vi "ProjectKFLOP.vi"() -> ()   [LabVIEW 2017]
uses:
  Control 1.ctl
  C:/KMotion434/KMotion/Release/KMotion_dotNet.dll
  Global 2.vi
panel:
  out "error out 3":errorcluster
  out "error out 2":errorcluster
  out "error out":errorcluster
  out "resulting string":string
  in  "Check_value":i32
  in  "BienLap":i32
  out "Status Check Done":dbl format="%11.1f"
  out "size":i32
  in  "Tab Control":enum32{"Manu", "Auto", "Setting"}(tab)
  in  "Add CheckDone":bool
  in  "Add Check":bool
  in  "Add Loop":bool
  in  "Test OUT":bool
  in  "Add Wait":bool
  in  "Add OUT":bool
  in  "TimeWait":dbl=5000.0
  in  "Value":dbl
  in  "Bit":dbl
  in  "Zero All":bool
  in  "Delele All":bool
  in  "Add Zero":bool
  in  "Add MoveXYZ":bool
  in  "Add Linear":bool
  in  "Save File":bool
  in  "Delete 1 Line":bool
  in  "Control":bool
  in  "Jog Speed":dbl=4000.0
  out "Vi Tri Save":string
  in  "file path (use dialog)":path
  out "Dest":dbl[](array[numeric])
  in  "Array Jog Command":dbl[](array[numeric])
  in  "V,A":dbl[](array[numeric]) caption="Dest 3"
  out "Auto":bool
  in  "Start":bool
  out "Value OUT":string
  out "Value Array":string[](array[string])
  out "Array":string[](array[string])
  out "Dest 2":T1
  out "Menu":bool
  in  "EMG":bool
  in  "Path":path
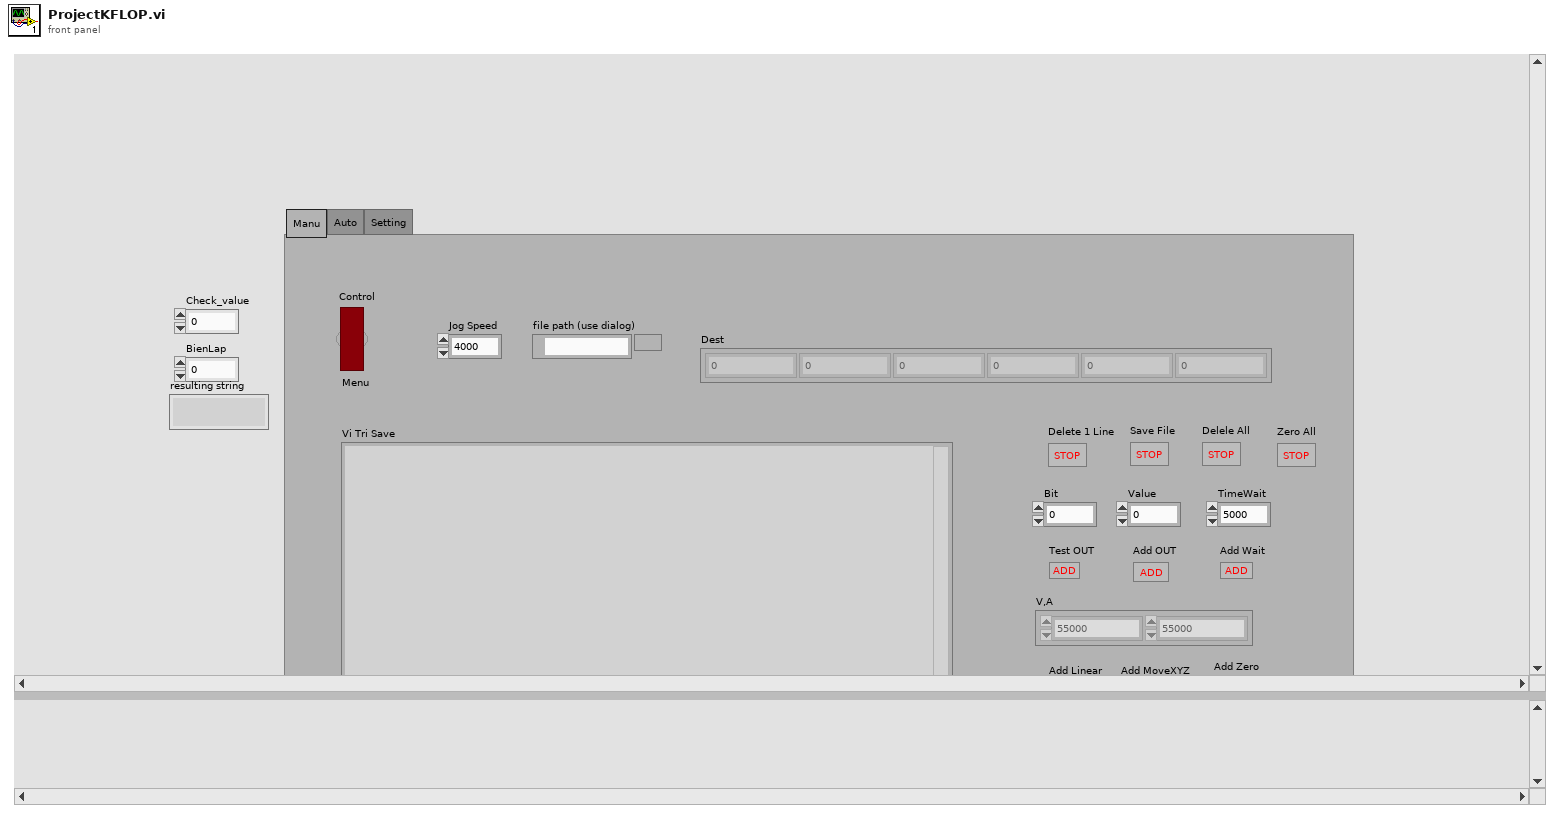
[diagram p1: front panel]
types:
  T1 = typedef "Control 1.ctl" = dbl[]
  T2 = cluster{"X":dbl, "Y":dbl, "Z":dbl, "A":dbl, "B":dbl, "C":dbl, "Numeric 7":dbl, "Numeric 8":dbl, "Numeric 9":dbl, "Numeric 10":dbl, "Numeric 11":dbl, "Numeric 12":dbl}
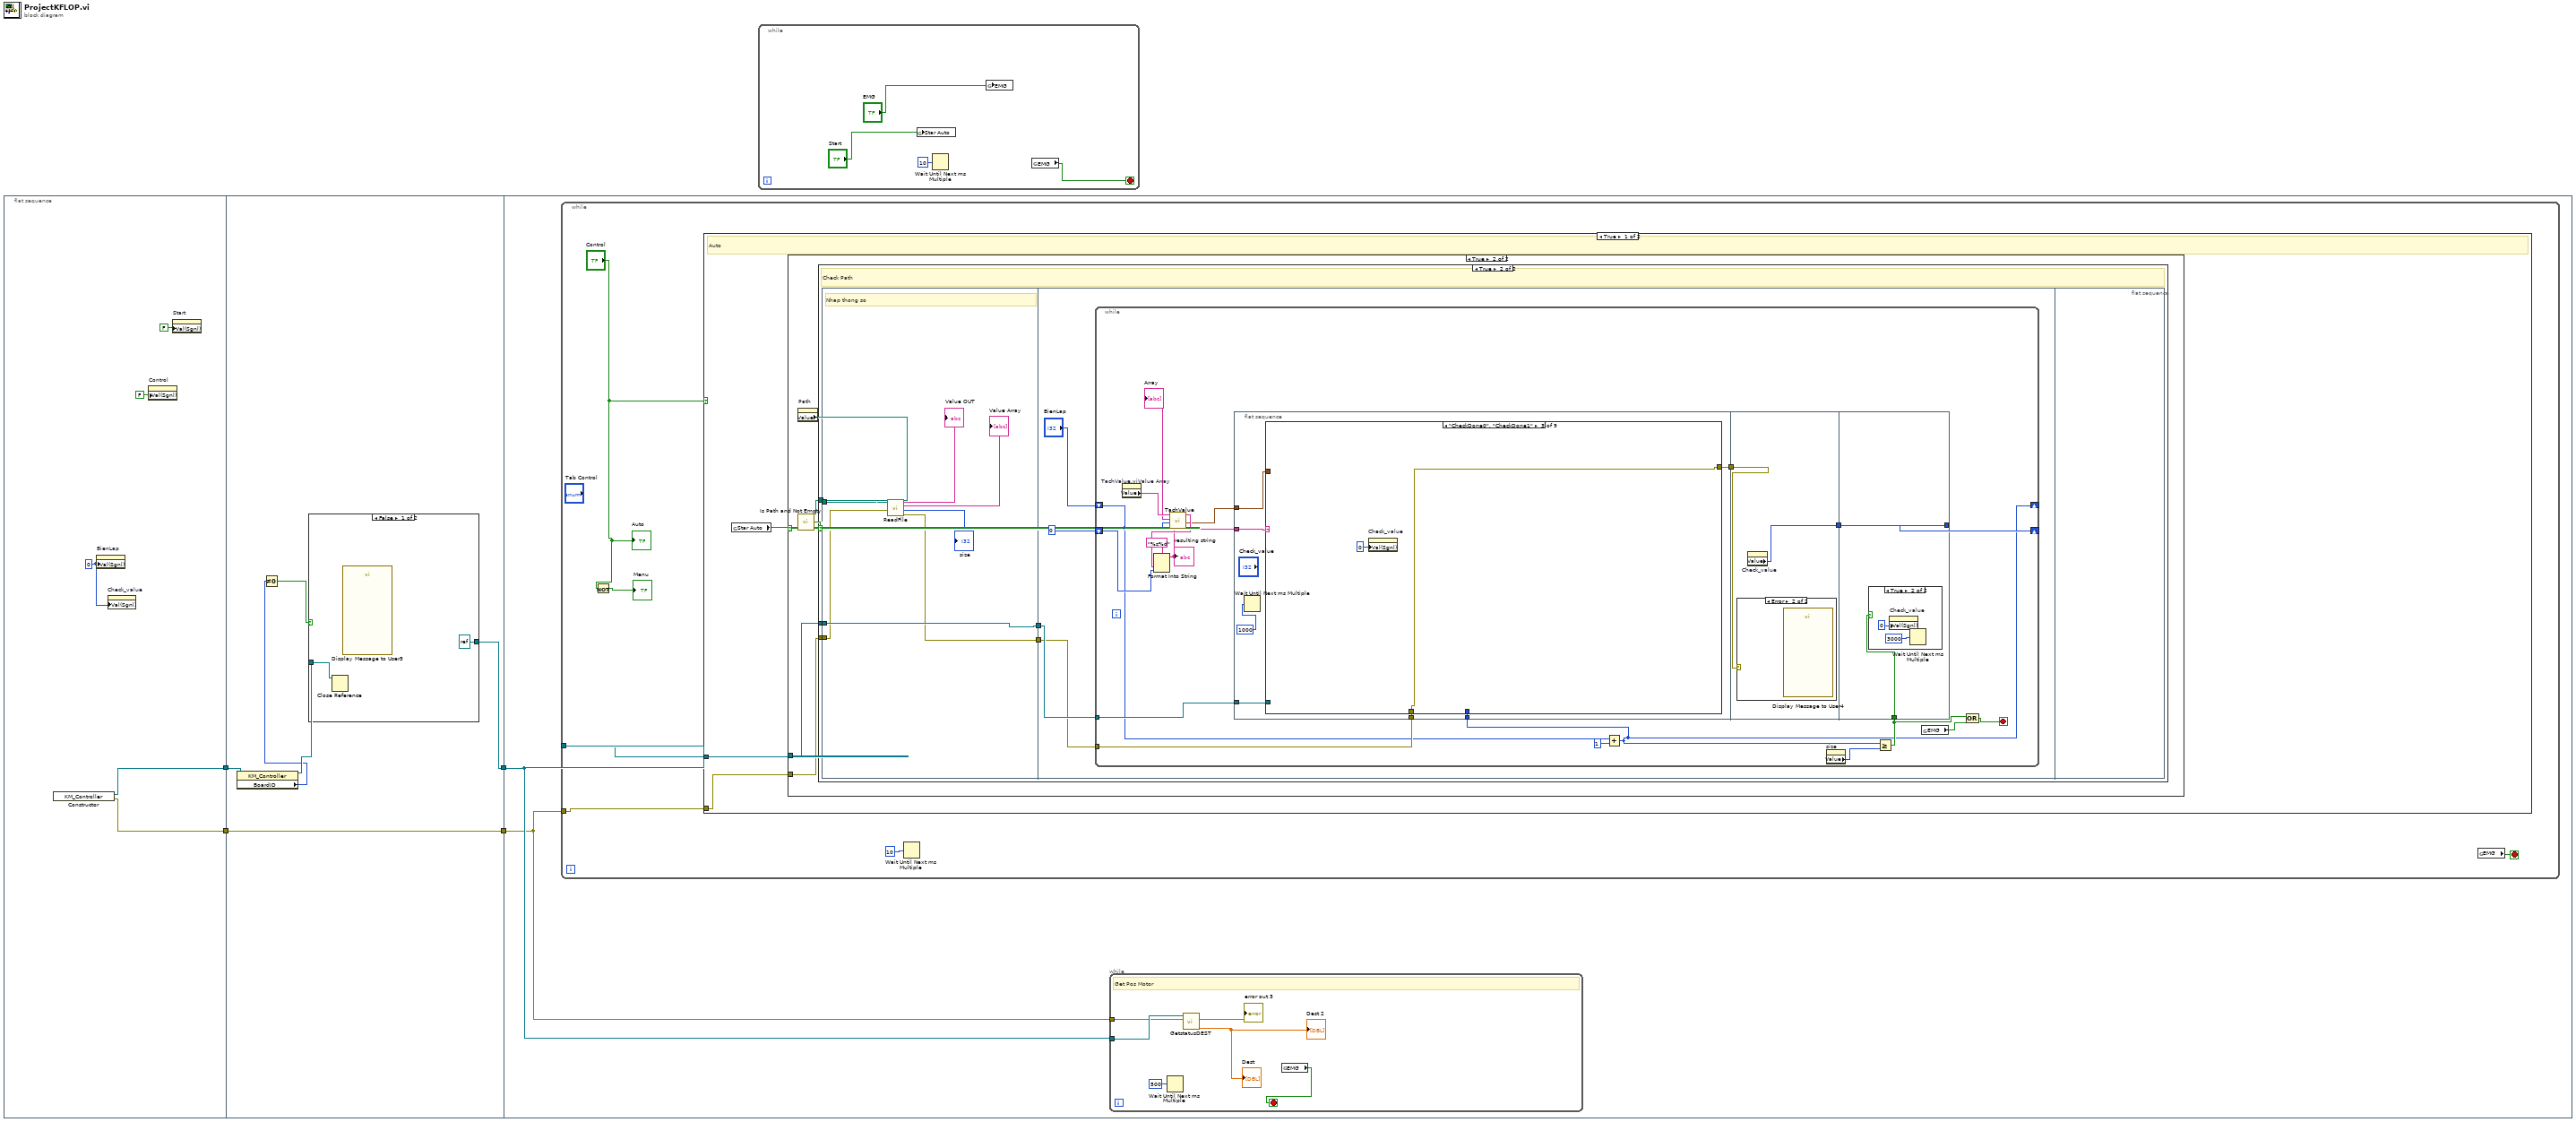
[diagram p0: block diagram]
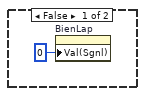
[diagram p3: hidden frame]
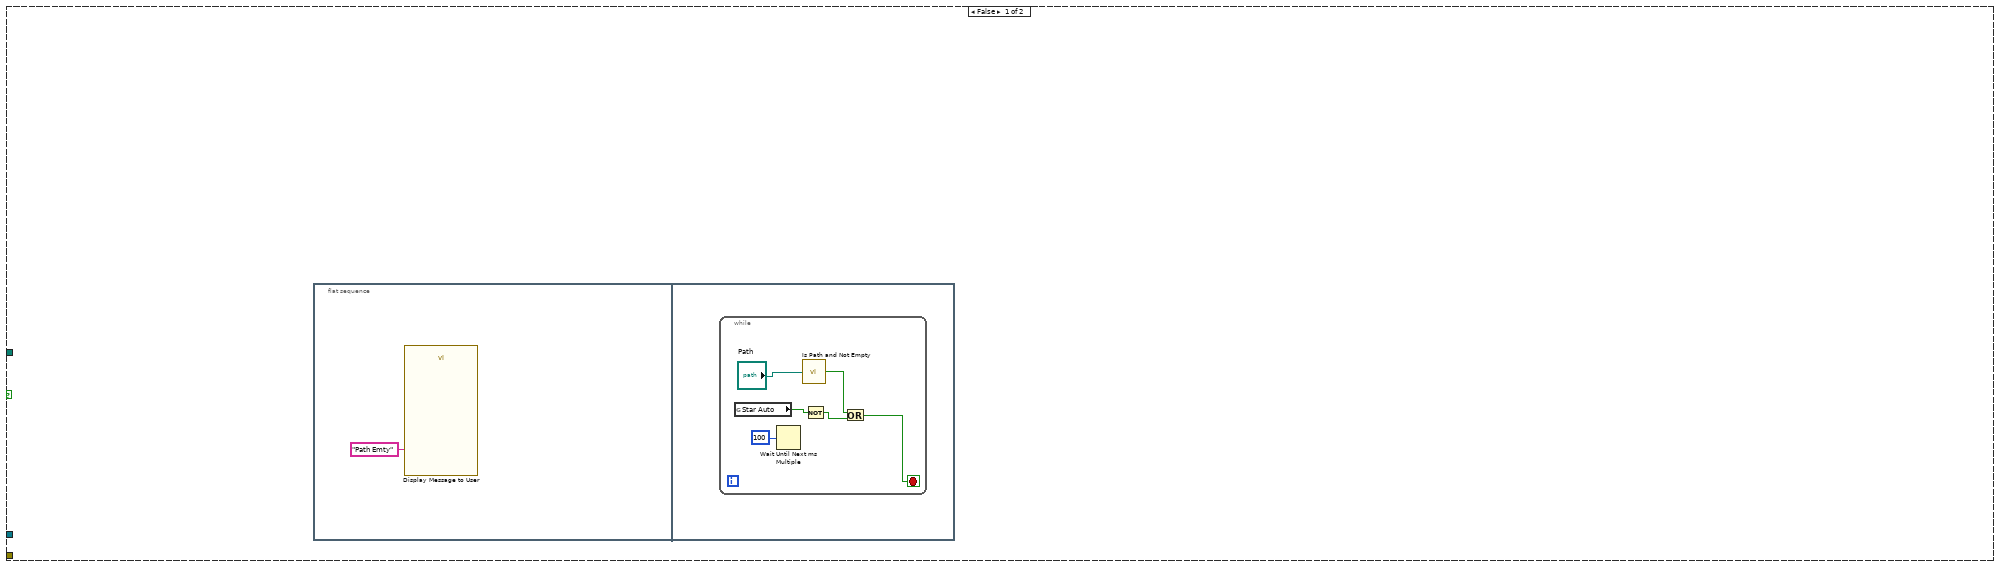
[diagram p4: hidden frame]
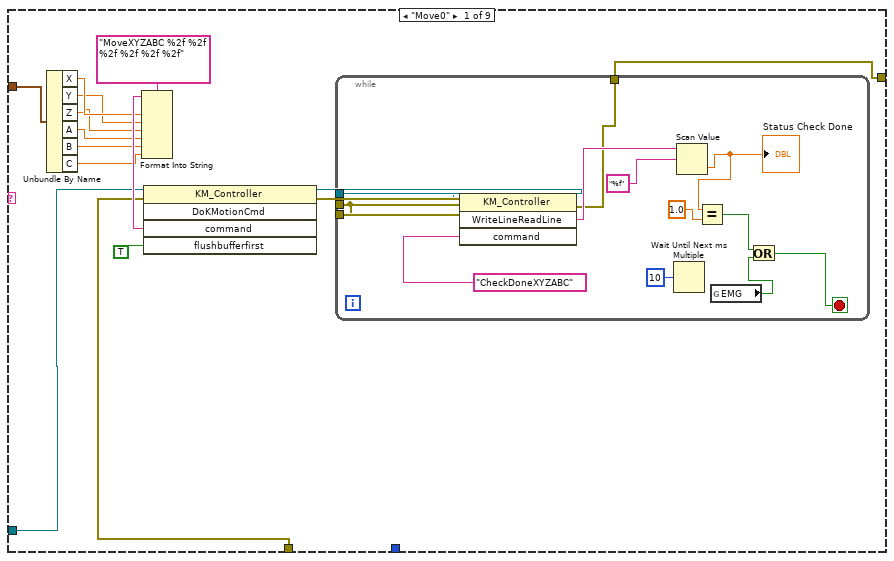
[diagram p5: hidden frame]
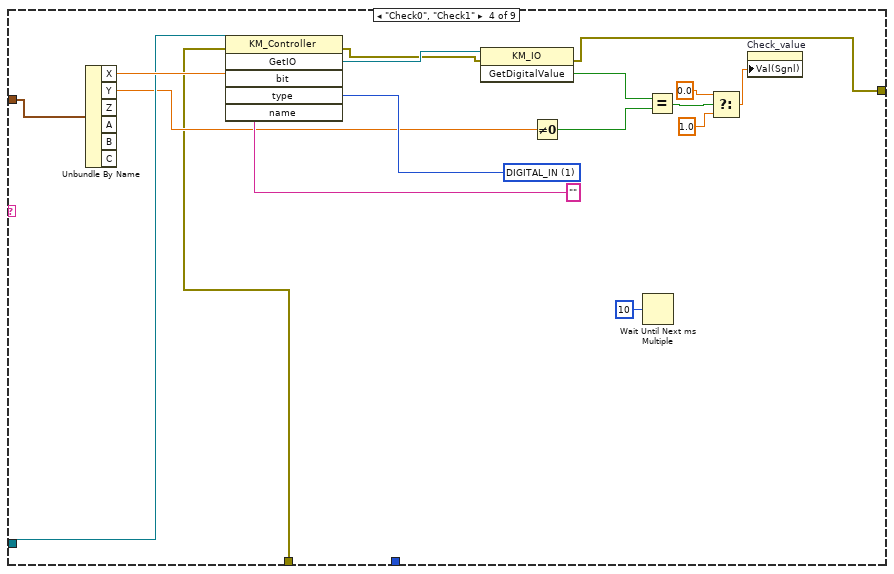
[diagram p7: hidden frame]
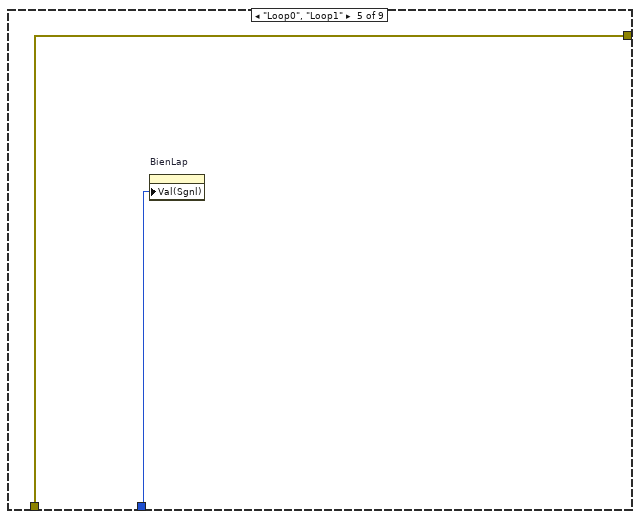
[diagram p8: hidden frame]
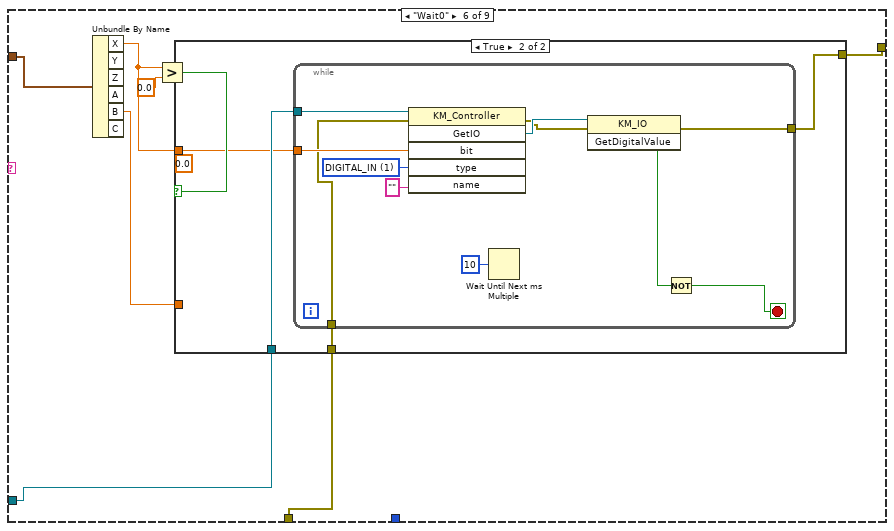
[diagram p9: hidden frame]
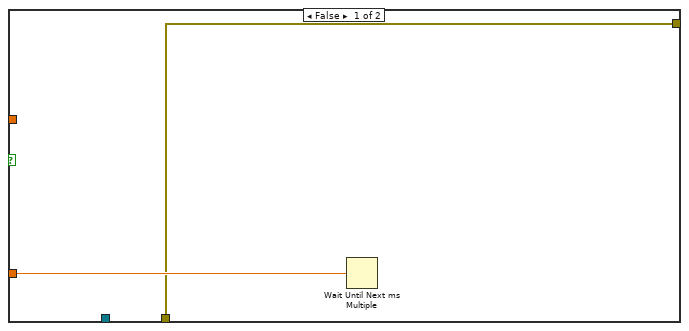
[diagram p10: hidden frame]
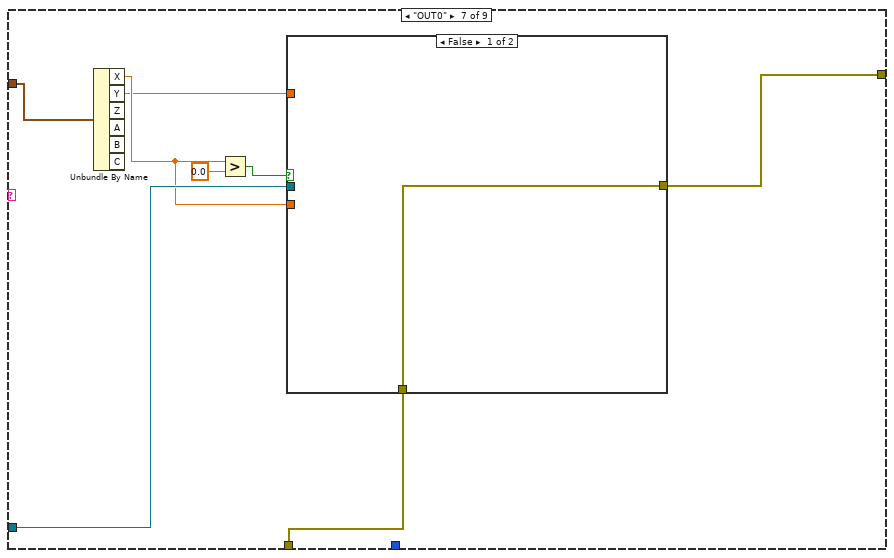
[diagram p11: hidden frame]
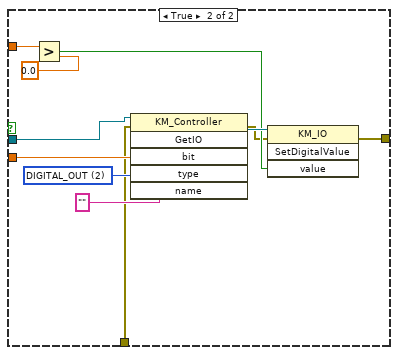
[diagram p12: hidden frame]
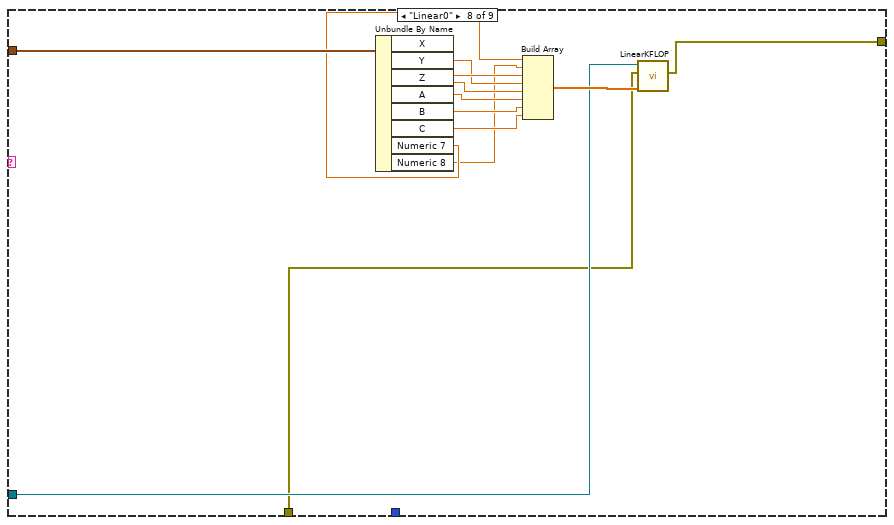
[diagram p13: hidden frame]
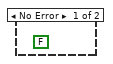
[diagram p15: hidden frame]
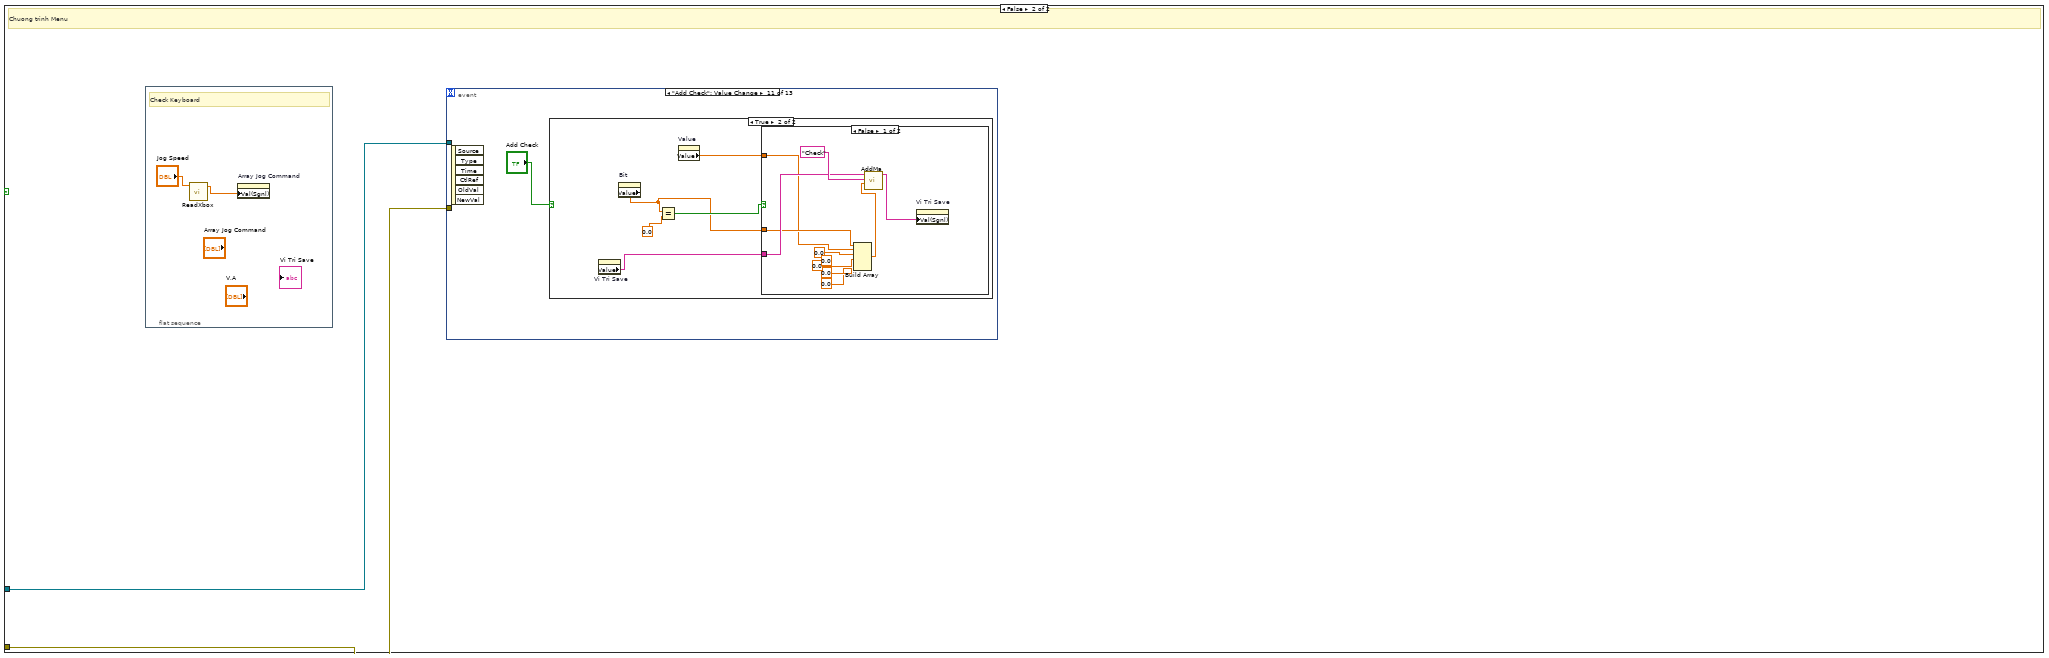
[diagram p17: hidden frame]
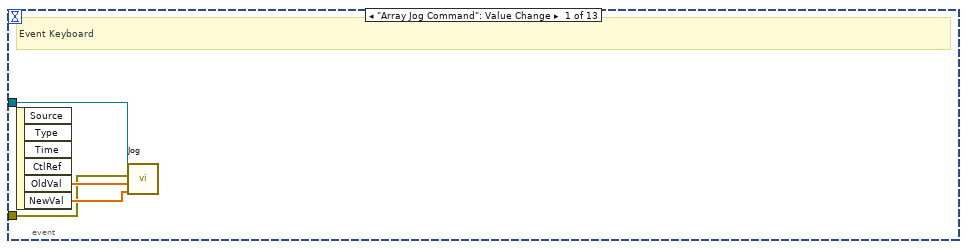
[diagram p18: hidden frame]
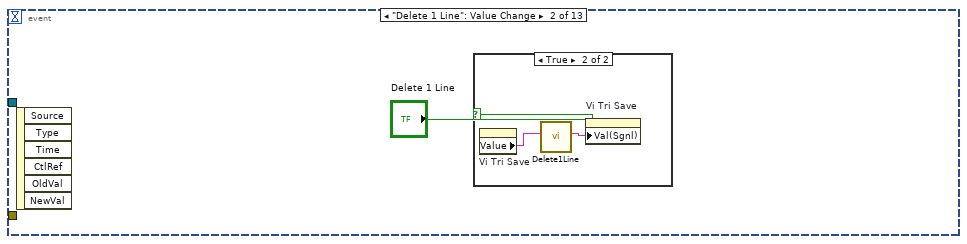
[diagram p19: hidden frame]
diagram:
  n1 = flat-sequence {
    tunnel: [w9] -> w2
    tunnel: [w8] -> w1
    tunnel: [w15] -> w4
    tunnel: [w14] -> w3
    tunnel: w2 -> [w13]
    tunnel: w1 -> [w15]
    tunnel: w4 -> [w19]
    tunnel: w3 -> [w20]
    frame #0 {
      w7 = 0 ("Value (Signaling)")
      n2 = constructor class="KM_Controller"() -> (reference out=w9:refnum<k24>, error out=w8:errorcluster)  [unwired: 3 in, 1 out]
      n3 = property on="BienLap" class="DigNum (strict)"("Val(Sgnl)"=w7) -> ()  [unwired: 2 in, 2 out]
      n4 = property on="Check_value" class="DigNum (strict)"("Val(Sgnl)"=w7) -> ()  [unwired: 2 in, 2 out]
      n5 = property on="Control" class="Bool (strict)"("Val(Sgnl)"=FALSE ("Value (Signaling)")) -> ()  [unwired: 2 in, 2 out]
      n6 = property on="Start" class="Bool (strict)"("Val(Sgnl)"=FALSE ("Value (Signaling)")) -> ()  [unwired: 2 in, 2 out]
    }
    frame #1 {
      n7 = property class="KM_Controller"(reference=w13) -> (reference out=w12:refnum<k24>, "BoardID"=w11:i32)  [unwired: 1 in, 1 out]
      n8 = Not Equal To 0?(x=w11) -> (x != 0?=w10:bool)
      n9 = case shown="False" w10 {
        tunnel: w12 -> [w16 w18]
        tunnel: [refnum<k24> refnum ("new reference") w18] -> w14
        frame False {
          n10 = Close Reference(reference=w16) -> ()  [unwired: 1 in, 1 out]
          n11 = call "Display Message to User3"() -> ()  [unwired: 10 in, 2 out]
        }
        frame True {
        }
      }
    }
    frame #2 {
      n12 = while {
        tunnel: w19 -> [w27]
        tunnel: w20 -> [w32]
        stop <- w28 stop-if-true
        n13 = Not(x="Control") -> (.not. x?=→"Menu":bool)
        n14 = case shown="True" "Control" {
          tunnel: w32 -> [w35 w204]
          tunnel: w27 -> [w33 w205]
          frame True {
            # "Auto"
            n15 = global read "Global 2.vi" "Star Auto"() -> (w34:bool)
            n16 = case shown="True" w34 {
              tunnel: w35 -> [_ w38]
              tunnel: w33 -> [_ w37]
              frame False {
                n17 = property on="BienLap" class="DigNum (strict)"("Val(Sgnl)"=0 ("Value (Signaling)")) -> ()  [unwired: 2 in, 2 out]
              }
              frame True {
                n18 = property on="Path" class="Path"() -> ("Value"=w39:path)  [unwired: 2 in, 2 out]
                n19 = call <vilib>:"Is Path and Not Empty.vi"("path"=w39) -> ("Is Path and Not Empty?"=w40:bool)  [unwired: 4 in]
                n20 = case shown="True" w40 {
                  tunnel: w39 -> [_ w51]
                  tunnel: w38 -> [_ w50]
                  tunnel: w37 -> [_ w49]
                  frame False {
                    n21 = flat-sequence {
                      frame #0 {
                        n22 = call "Display Message to User"("Message"="Path Emty") -> ()  [unwired: 9 in, 2 out]
                      }
                      frame #1 {
                        n23 = while {
                          stop <- w45 stop-if-true
                          n24 = global read "Global 2.vi" "Star Auto"() -> (w42:bool)
                          n25 = Wait Until Next ms Multiple(millisecond multiple=u32 100) -> ()  [unwired: 1 out]
                          n26 = call <vilib>:"Is Path and Not Empty.vi"("path"="Path") -> ("Is Path and Not Empty?"=w44:bool)  [unwired: 4 in]
                          n27 = Not(x=w42) -> (.not. x?=w43:bool)
                          n28 = Or(x=w44, y=w43) -> (x .or. y?=w45:bool)
                        }
                      }
                    }
                  }
                  frame True {
                    # "Check Path"
                    n29 = flat-sequence {
                      tunnel: [w55] -> w52
                      tunnel: w51 -> [w57]
                      tunnel: w50 -> [w55]
                      tunnel: w49 -> [w54]
                      tunnel: [w53] -> w48
                      tunnel: w52 -> [w63]
                      tunnel: w48 -> [w61]
                      frame #0 {
                        # "Nhap thong so"
                        n30 = call "ReadFile.vi"("error in"=w54, "Path"=w57) -> ("error out"=w53:errorcluster, "size"=→"size":i32, "Value Array"=→"Value Array":string[], "Value OUT"=→"Value OUT":string)  [unwired: 6 in]
                      }
                      frame #1 {
                        n31 = while {
                          shift-right: [w64] -> _
                          shift-left: "BienLap" -> [w65]
                          shift-right: [w70] -> _
                          shift-left: 0 -> [w79]
                          tunnel: w63 -> [w73]
                          tunnel: w61 -> [w72]
                          stop <- w75 stop-if-true
                          n32 = property on="TachValue.viValue Array" class="Arr (strict)"() -> ("Value"=w82:string[])  [unwired: 2 in, 2 out]
                          n33 = call "TachValue.vi"("index"=w65, "array"=w82) -> ("Cluster"=w69:T2, "Array"=→"Array":string[], "OUT First Value"=w77:string)  [unwired: 7 in]
                          n34 = Format Into String(format string="%s%d", w77, w79) -> (resulting string=w74:string)  [unwired: 2 in, 1 out]
                          "resulting string" <- w74
                          n35 = flat-sequence {
                            tunnel: w74 -> [w89]
                            tunnel: w69 -> [w88]
                            tunnel: w73 -> [w87]
                            tunnel: w72 -> [w86]
                            tunnel: [w85] -> w71
                            tunnel: w64 -> [w83]
                            tunnel: w71 -> [w199]
                            tunnel: [w198] -> w68
                            tunnel: [w201] -> w70
                            tunnel: w68 -> [w201]
                            tunnel: w67 -> [w200]
                            frame #0 {
                              n36 = Wait Until Next ms Multiple(millisecond multiple=u32 1000) -> ()  [unwired: 1 out]
                              n37 = case shown="\"CheckDone0\", \"CheckDone1\"" w89 {
                                tunnel: w88 -> [w99 _ _ w134 _ w146 w171 w196 _]
                                tunnel: w87 -> [w92 _ _ w135 _ w143 w168 w188 _]
                                tunnel: [w91 w117 w118 w121 w138 w139 w165 w185 w197] -> w85
                                tunnel: w86 -> [w90 w117 w118 w120 w138 w140 w164 w184 w197]
                                tunnel: w83 -> [_ _ _ _ w137 _ _ _ _]
                                frame "Move0" {
                                n38 = Unbundle By Name(w99) -> ("X"=w98:dbl, "Y"=w97:dbl, "Z"=w96:dbl, "A"=w95:dbl, "B"=w94:dbl, "C"=w93:dbl)
                                n39 = Format Into String(format string="MoveXYZABC %2f %2f %2f %2f %2f %2f", w98, w97, w96, w95, w94, w93) -> (resulting string=w102:string)  [unwired: 2 in, 1 out]
                                n40 = invoke class="KM_Controller" method="DoKMotionCmd"(reference=w92, error in=w90, "command"=w102, "flushbufferfirst"=TRUE) -> (reference out=w101:refnum<k24>, error out=w100:errorcluster)  [unwired: 1 in, 3 out]
                                n41 = while {
                                tunnel: [w107] -> _
                                tunnel: w101 -> [w108]
                                tunnel: w100 -> [w107]
                                tunnel: [w105] -> w91
                                stop <- w110 stop-if-true
                                n42 = invoke class="KM_Controller" method="WriteLineReadLine"(reference=w108, error in=w107, "command"="CheckDoneXYZABC") -> (error out=w105:errorcluster, "WriteLineReadLine"=w116:string)  [unwired: 1 in, 2 out]
                                n43 = Wait Until Next ms Multiple(millisecond multiple=u32 10) -> ()  [unwired: 1 out]
                                n44 = Scan Value(string=w116, format string="%f") -> (value=w113:dbl)  [unwired: 1 in, 1 out]
                                "Status Check Done" <- w113
                                n45 = Equal?(x=w113, y=1.0 ("x")) -> (x = y?=w109:bool)
                                n46 = global read "Global 2.vi" "EMG"() -> (w106:bool)
                                n47 = Or(x=w109, y=w106) -> (x .or. y?=w110:bool)
                                }
                                }
                                frame Default {
                                }
                                frame "CheckDone0", "CheckDone1" {
                                n48 = property on="Check_value" class="DigNum (strict)"("Val(Sgnl)"=0 ("Value (Signaling)")) -> ()  [unwired: 2 in, 2 out]
                                }
                                frame "Check0", "Check1" {
                                w133 = 1 items=["UNDEFINED", "DIGITAL_IN", "DIGITAL_OUT", "ANALOG_IN", "ANALOG_OUT"] ("type")
                                n49 = Unbundle By Name(w134) -> ("X"=w136:dbl, "Y"=w128:dbl)  [unwired: 4 out]
                                n50 = invoke class="KM_Controller" method="GetIO"(reference=w135, error in=w120, "bit"=w136, "type"=w133, "name"="") -> (error out=w122:errorcluster, "GetIO"=w132:refnum<k24>)  [unwired: 1 in, 4 out]
                                n51 = invoke class="KM_IO" method="GetDigitalValue"(reference=w132, error in=w122) -> (error out=w121:errorcluster, "GetDigitalValue"=w129:bool)  [unwired: 1 in, 1 out]
                                n52 = Not Equal To 0?(x=w128) -> (x != 0?=w127:bool)
                                n53 = Wait Until Next ms Multiple(millisecond multiple=u32 10) -> ()  [unwired: 1 out]
                                n54 = Equal?(x=w129, y=w127) -> (x = y?=w123:bool)
                                n55 = Select(t=0.0, s=w123, f=1.0) -> (s? t:f=w126:dbl)
                                n56 = property on="Check_value" class="DigNum (strict)"("Val(Sgnl)"=w126) -> ()  [unwired: 2 in, 2 out]
                                }
                                frame "Loop0", "Loop1" {
                                n57 = property on="BienLap" class="DigNum (strict)"("Val(Sgnl)"=w137) -> ()  [unwired: 2 in, 2 out]
                                }
                                frame "Wait0" {
                                n58 = Unbundle By Name(w146) -> ("X"=w142:dbl, "B"=w145:dbl)  [unwired: 4 out]
                                n59 = Greater?(x=w142, y=0.0) -> (0:w141:bool)
                                n60 = case shown="True" w141 {
                                tunnel: w145 -> [w148 _]
                                tunnel: w143 -> [_ w152]
                                tunnel: w142 -> [_ w151]
                                tunnel: [w147 w150] -> w139
                                tunnel: w140 -> [w147 w149]
                                frame False {
                                n61 = Wait Until Next ms Multiple(millisecond multiple=w148) -> ()  [unwired: 1 out]
                                }
                                frame True {
                                (unwired) 0.0 ("y")
                                n62 = while {
                                tunnel: w152 -> [w163]
                                tunnel: w151 -> [w161]
                                tunnel: [w154] -> w150
                                tunnel: w149 -> [w153]
                                stop <- w158 stop-if-true
                                w162 = 1 items=["UNDEFINED", "DIGITAL_IN", "DIGITAL_OUT", "ANALOG_IN", "ANALOG_OUT"] ("type")
                                n63 = invoke class="KM_Controller" method="GetIO"(reference=w163, error in=w153, "bit"=w161, "type"=w162, "name"="") -> (error out=w155:errorcluster, "GetIO"=w160:refnum<k24>)  [unwired: 1 in, 4 out]
                                n64 = Wait Until Next ms Multiple(millisecond multiple=u32 10) -> ()  [unwired: 1 out]
                                n65 = invoke class="KM_IO" method="GetDigitalValue"(reference=w160, error in=w155) -> (error out=w154:errorcluster, "GetDigitalValue"=w157:bool)  [unwired: 1 in, 1 out]
                                n66 = Not(x=w157) -> (.not. x?=w158:bool)
                                }
                                }
                                }
                                }
                                frame "OUT0" {
                                n67 = Unbundle By Name(w171) -> ("X"=w167:dbl, "Y"=w166:dbl)  [unwired: 4 out]
                                n68 = Greater?(x=w167, y=0.0) -> (0:w170:bool)
                                n69 = case shown="False" w170 {
                                tunnel: w168 -> [_ w176]
                                tunnel: w167 -> [_ w177]
                                tunnel: w166 -> [_ w180]
                                tunnel: [w172 w174] -> w165
                                tunnel: w164 -> [w172 w173]
                                frame False {
                                }
                                frame True {
                                w183 = 2 items=["UNDEFINED", "DIGITAL_IN", "DIGITAL_OUT", "ANALOG_IN", "ANALOG_OUT"] ("type")
                                n70 = Greater?(x=w180, y=0.0) -> (0:w179:bool)
                                n71 = invoke class="KM_Controller" method="GetIO"(reference=w176, error in=w173, "bit"=w177, "type"=w183, "name"="") -> (error out=w175:errorcluster, "GetIO"=w181:refnum<k24>)  [unwired: 1 in, 4 out]
                                n72 = invoke class="KM_IO" method="SetDigitalValue"(reference=w181, error in=w175, "value"=w179) -> (error out=w174:errorcluster)  [unwired: 1 in, 3 out]
                                }
                                }
                                }
                                frame "Linear0" {
                                n73 = Unbundle By Name(w196) -> ("X"=w195:dbl, "Y"=w194:dbl, "Z"=w193:dbl, "A"=w192:dbl, "B"=w191:dbl, "C"=w190:dbl, "Numeric 7"=w187:dbl, "Numeric 8"=w186:dbl)
                                n74 = Build Array(w187, w186, w195, w194, w193, w192, w191, w190) -> (w189:dbl[])
                                n75 = call "LinearKFLOP.vi"("Array"=w189, "error in (no error)"=w184, "new reference"=w188) -> ("error out"=w185:errorcluster)  [unwired: 7 in, 1 out]
                                }
                                frame "M010" {
                                }
                              }
                            }
                            frame #1 {
                              n76 = case shown="Error" w199 {
                                frame No Error {
                                (unwired) FALSE ("OK")
                                }
                                frame Error {
                                n77 = call "Display Message to User4"() -> ()  [unwired: 10 in, 2 out]
                                }
                              }
                              n78 = property on="Check_value" class="DigNum (strict)"() -> ("Value"=w198:i32)  [unwired: 2 in, 2 out]
                            }
                            frame #2 {
                              n79 = case shown="True" w200 {
                                frame False {
                                }
                                frame True {
                                n80 = property on="Check_value" class="DigNum (strict)"("Val(Sgnl)"=0 ("Value (Signaling)")) -> ()  [unwired: 2 in, 2 out]
                                n81 = Wait Until Next ms Multiple(millisecond multiple=u32 3000) -> ()  [unwired: 1 out]
                                }
                              }
                            }
                          }
                          n82 = Add(x=w65, y=1) -> (x+y=w64:i32)
                          n83 = property on="size" class="DigNum (strict)"() -> ("Value"=w66:i32)  [unwired: 2 in, 2 out]
                          n84 = Greater Or Equal?(x=w64, y=w66) -> (x >= y?=w67:bool)
                          n85 = global read "Global 2.vi" "EMG"() -> (w76:bool)
                          n86 = Compound Arithmetic op=OR(w67, w76) -> (w75:bool)
                        }
                      }
                      frame #2 {
                      }
                    }
                  }
                }
              }
            }
          }
          frame False {
            # "Chuong trinh Menu"
            n87 = flat-sequence {
              frame #0 {
                # "Check Keyboard"
                n88 = call "ReadXbox.vi"("Jog Speed"="Jog Speed") -> ("Array Jog Command"=w312:dbl[])  [unwired: 5 in]
                n89 = property on="Array Jog Command" class="Arr (strict)"("Val(Sgnl)"=w312) -> ()  [unwired: 2 in, 2 out]
              }
            }
            n90 = event shown="[10] \"Add Check\": Value Change" {
              selector: _ -> [_ _ _ _ _ _ _ _ _ _ _ _ _]
              dyn-events: _ -> [_ _ _ _ _ _ _ _ _ _ _ _ _]
              timeout: _ -> [_ _ _ _ _ _ _ _ _ _ _ _ _]
              tunnel: w204 -> [w207 _ _ _ w218 w234 _ _ _ _ _ _ _]
              tunnel: w205 -> [w206 _ _ _ w219 w232 _ _ _ _ _ _ _]
              event "Array Jog Command": Value Change {
                # "Event Keyboard"
                n91 = event-data() -> ("OldVal"=w209:dbl[], "NewVal"=w208:dbl[])  [unwired: 1 in, 4 out]
                n92 = call "Jog.vi"("NewVal"=w208, "Old Var"=w209, "error in (no error)"=w206, "reference"=w207) -> ()  [unwired: 6 in, 2 out]
              }
              event "Delete 1 Line": Value Change {
                n93 = event-data() -> ()  [unwired: 1 in, 6 out]
                n94 = case shown="True" "Delete 1 Line" {
                  frame False {
                  }
                  frame True {
                    n95 = property on="Vi Tri Save" class="Str"() -> ("Value"=w212:string)  [unwired: 2 in, 2 out]
                    n96 = call "Delete1Line.vi"("Value"=w212) -> ("String"=w211:string)  [unwired: 10 in]
                    n97 = property on="Vi Tri Save" class="Str"("Val(Sgnl)"=w211) -> ()  [unwired: 2 in, 2 out]
                  }
                }
              }
              event "Delele All": Value Change {
                n98 = event-data() -> ()  [unwired: 1 in, 6 out]
                n99 = case shown="True" "Delele All" {
                  frame False {
                  }
                  frame True {
                    n100 = property on="Vi Tri Save" class="Str"("Val(Sgnl)"="" ("Value (Signaling)")) -> ()  [unwired: 2 in, 2 out]
                  }
                }
              }
              event "Save File": Value Change {
                n101 = event-data() -> ()  [unwired: 1 in, 6 out]
                n102 = case shown="True" "Save File" {
                  frame False {
                  }
                  frame True {
                    n103 = property on="Vi Tri Save" class="Str"() -> ("Value"=w216:string)  [unwired: 2 in, 2 out]
                    n104 = call "SaveFile.vi"("text"=w216, "file path (use dialog)"="file path (use dialog)") -> ()  [unwired: 10 in]
                  }
                }
              }
              event "Test OUT": Value Change {
                n105 = event-data() -> ()  [unwired: 1 in, 6 out]
                n106 = case shown="True" "Test OUT" {
                  tunnel: w218 -> [_ w224]
                  tunnel: w219 -> [_ w223]
                  frame False {
                  }
                  frame True {
                    w231 = 2 items=["UNDEFINED", "DIGITAL_IN", "DIGITAL_OUT", "ANALOG_IN", "ANALOG_OUT"] ("type")
                    n107 = property on="Value" class="DigNum (strict)"() -> ("Value"=w226:dbl)  [unwired: 2 in, 2 out]
                    n108 = Greater?(x=w226, y=0.0) -> (0:w228:bool)
                    n109 = property on="Bit" class="DigNum (strict)"() -> ("Value"=w225:dbl)  [unwired: 2 in, 2 out]
                    n110 = invoke class="KM_Controller" method="GetIO"(reference=w224, error in=w223, "bit"=w225, "type"=w231, "name"="") -> (error out=w222:errorcluster, "GetIO"=w229:refnum<k24>)  [unwired: 1 in, 4 out]
                    n111 = invoke class="KM_IO" method="SetDigitalValue"(reference=w229, error in=w222, "value"=w228) -> (error out=→"error out":errorcluster)  [unwired: 1 in, 3 out]
                  }
                }
              }
              event "Zero All": Value Change {
                n112 = event-data() -> ()  [unwired: 1 in, 6 out]
                n113 = case shown="True" "Zero All" {
                  tunnel: w234 -> [_ w237]
                  tunnel: w232 -> [_ w236]
                  frame False {
                  }
                  frame True {
                    n114 = call "SetZeroALL.vi"("error in (no error)"=w236, "reference"=w237) -> ("error out"=→"error out 2":errorcluster)  [unwired: 8 in, 1 out]
                  }
                }
              }
              event "Add Zero": Value Change {
                n115 = event-data() -> ()  [unwired: 1 in, 6 out]
                n116 = case shown="True" "Add Zero" {
                  frame False {
                  }
                  frame True {
                    n117 = property on="V,A" class="Arr (strict)"() -> ("Value"=w240:dbl[])  [unwired: 2 in, 2 out]
                    n118 = property on="Vi Tri Save" class="Str"() -> ("Value"=w242:string)  [unwired: 2 in, 2 out]
                    n119 = call "AddMa.vi"("Dest 3"=w240, "Toa Do"=dbl[] [], "MaBegin"="Linear", "String IN"=w242) -> ("String OUT"=w241:string)  [unwired: 7 in]
                    n120 = property on="Vi Tri Save" class="Str"("Val(Sgnl)"=w241) -> ()  [unwired: 2 in, 2 out]
                  }
                }
              }
              event "Add OUT": Value Change {
                n121 = event-data() -> ()  [unwired: 1 in, 6 out]
                n122 = property on="Bit" class="DigNum (strict)"() -> ("Value"=w246:dbl)  [unwired: 2 in, 2 out]
                n123 = case shown="True" "Add OUT" {
                  tunnel: w246 -> [_ w252]
                  tunnel: "Value" -> [_ w251]
                  frame False {
                  }
                  frame True {
                    n124 = Build Array(w252, w251, 0.0 ("element"), 0.0 ("element"), 0.0 ("element"), 0.0 ("element")) -> (w255:dbl[])
                    n125 = property on="Vi Tri Save" class="Str"() -> ("Value"=w253:string)  [unwired: 2 in, 2 out]
                    n126 = call "AddMa.vi"("Toa Do"=w255, "MaBegin"="OUT", "String IN"=w253) -> ("String OUT"=w254:string)  [unwired: 8 in]
                    n127 = property on="Vi Tri Save" class="Str"("Val(Sgnl)"=w254) -> ()  [unwired: 2 in, 2 out]
                  }
                }
              }
              event "Add Wait": Value Change {
                n128 = event-data() -> ()  [unwired: 1 in, 6 out]
                n129 = case shown="True" "Add Wait" {
                  tunnel: "Bit" -> [_ w265]
                  tunnel: "TimeWait" -> [_ w264]
                  frame False {
                  }
                  frame True {
                    n130 = Build Array(w265, 0.0 ("element"), 0.0 ("element"), 0.0 ("element"), w264, 0.0 ("element")) -> (w266:dbl[])
                    n131 = property on="Vi Tri Save" class="Str"() -> ("Value"=w269:string)  [unwired: 2 in, 2 out]
                    n132 = call "AddMa.vi"("Toa Do"=w266, "MaBegin"="Wait", "String IN"=w269) -> ("String OUT"=w268:string)  [unwired: 8 in]
                    n133 = property on="Vi Tri Save" class="Str"("Val(Sgnl)"=w268) -> ()  [unwired: 2 in, 2 out]
                  }
                }
              }
              event "Add Loop": Value Change {
                n134 = event-data() -> ()  [unwired: 1 in, 6 out]
                n135 = case shown="True" "Add Loop" {
                  frame False {
                  }
                  frame True {
                    n136 = property on="Vi Tri Save" class="Str"() -> ("Value"=w279:string)  [unwired: 2 in, 2 out]
                    n137 = Build Array(0.0 ("element"), 0.0 ("element"), 0.0 ("element"), 0.0 ("element"), 0.0 ("element"), 0.0 ("element")) -> (w271:dbl[])
                    n138 = call "AddMa.vi"("Toa Do"=w271, "MaBegin"="Loop", "String IN"=w279) -> ("String OUT"=w280:string)  [unwired: 8 in]
                    n139 = property on="Vi Tri Save" class="Str"("Val(Sgnl)"=w280) -> ()  [unwired: 2 in, 2 out]
                  }
                }
              }
              event "Add Check": Value Change {
                n140 = event-data() -> ()  [unwired: 1 in, 6 out]
                n141 = case shown="True" "Add Check" {
                  frame False {
                  }
                  frame True {
                    n142 = property on="Vi Tri Save" class="Str"() -> ("Value"=w282:string)  [unwired: 2 in, 2 out]
                    n143 = property on="Bit" class="DigNum (strict)"() -> ("Value"=w284:dbl)  [unwired: 2 in, 2 out]
                    n144 = Equal?(x=w284, y=0.0) -> (x = y?=w285:bool)
                    n145 = property on="Value" class="DigNum (strict)"() -> ("Value"=w283:dbl)  [unwired: 2 in, 2 out]
                    n146 = case shown="False" w285 {
                      tunnel: w282 -> [w291 _]
                      tunnel: w284 -> [w289 _]
                      tunnel: w283 -> [w288 _]
                      frame False {
                        (unwired) 0.0 ("element")
                        n147 = Build Array(w289, w288, 0.0 ("element"), 0.0 ("element"), 0.0 ("element"), 0.0 ("element")) -> (w287:dbl[])
                        n148 = call "AddMa.vi"("Toa Do"=w287, "MaBegin"="Check", "String IN"=w291) -> ("String OUT"=w290:string)  [unwired: 8 in]
                        n149 = property on="Vi Tri Save" class="Str"("Val(Sgnl)"=w290) -> ()  [unwired: 2 in, 2 out]
                      }
                      frame True {
                        n150 = call "Display Message to User2"() -> ()  [unwired: 10 in, 2 out]
                      }
                    }
                  }
                }
              }
              event "Add CheckDone": Value Change {
                n151 = event-data() -> ()  [unwired: 1 in, 6 out]
                n152 = case shown="True" "Add CheckDone" {
                  frame False {
                  }
                  frame True {
                    n153 = property on="Vi Tri Save" class="Str"() -> ("Value"=w299:string)  [unwired: 2 in, 2 out]
                    n154 = call "AddMa.vi"("MaBegin"="CheckDone", "String IN"=w299) -> ("String OUT"=w300:string)  [unwired: 9 in]
                    n155 = property on="Vi Tri Save" class="Str"("Val(Sgnl)"=w300) -> ()  [unwired: 2 in, 2 out]
                  }
                }
              }
              event "Add Linear", "Add MoveXYZ": Value Change {
                n156 = event-data() -> ()  [unwired: 1 in, 6 out]
                n157 = Select(t="Move", s="Add MoveXYZ", f="Linear") -> (s? t:f=w301:string)
                n158 = Or(x="Add Linear", y="Add MoveXYZ") -> (x .or. y?=w302:bool)
                n159 = case shown="True" w302 {
                  tunnel: w301 -> [_ w308]
                  frame False {
                  }
                  frame True {
                    n160 = property on="Vi Tri Save" class="Str"() -> ("Value"=w310:string)  [unwired: 2 in, 2 out]
                    n161 = property on="Dest" class="Arr (strict)"() -> ("Value"=w309:dbl[])  [unwired: 2 in, 2 out]
                    n162 = property on="V,A" class="Arr (strict)"() -> ("Value"=w307:dbl[])  [unwired: 2 in, 2 out]
                    n163 = call "AddMa.vi"("Dest 3"=w307, "Toa Do"=w309, "MaBegin"=w308, "String IN"=w310) -> ("String OUT"=w311:string)  [unwired: 7 in]
                    n164 = property on="Vi Tri Save" class="Str"("Val(Sgnl)"=w311) -> ()  [unwired: 2 in, 2 out]
                  }
                }
              }
            }
          }
        }
        n165 = Wait Until Next ms Multiple(millisecond multiple=u32 10) -> ()  [unwired: 1 out]
        n166 = global read "Global 2.vi" "EMG"() -> (w28:bool)
        "Auto" <- "Control"
      }
      n167 = while {
        tunnel: w20 -> [w25]
        tunnel: w19 -> [w22]
        stop <- w23 stop-if-true
        # "Get Pos Motor"
        n168 = Wait Until Next ms Multiple(millisecond multiple=u32 500) -> ()  [unwired: 1 out]
        n169 = call "GetstatusDEST.vi"("error in (no error)"=w22, "new reference"=w25) -> ("Dest"=→"Dest" →"Dest 2":dbl[], "error out"=→"error out 3":errorcluster)  [unwired: 7 in, 1 out]
        n170 = global read "Global 2.vi" "EMG"() -> (w23:bool)
      }
    }
  }
  n171 = while {
    stop <- w316 stop-if-true
    n172 = global write "Global 2.vi" "Star Auto"("Start") -> ()
    n173 = Wait Until Next ms Multiple(millisecond multiple=u32 10) -> ()  [unwired: 1 out]
    n174 = global write "Global 2.vi" "EMG"("EMG") -> ()
    n175 = global read "Global 2.vi" "EMG"() -> (w316:bool)
  }
